vi "CPU_SP_push.vi"(10 "value":u8 format="%02x", 11 "registers":T1 {"P" format="%08b"; "PC" format="%04x"; "SP" format="%02x"; "Y" format="%02x"; "X" format="%02x"; "A" format="%02x"}) -> (3 "registers":T1 {"P" format="%08b"; "PC" format="%04x"; "SP" format="%02x"; "Y" format="%02x"; "X" format="%02x"; "A" format="%02x"})   [LabVIEW 2018]
uses:
  CPU_registers.ctl
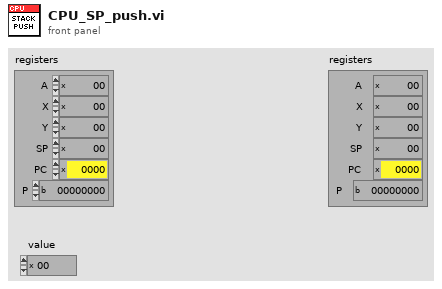
[diagram p1: front panel]
types:
  T1 = typedef "CPU_registers.ctl" = cluster{"A":u8, "X":u8, "Y":u8, "SP":u8, "PC":u16, "P":u8}
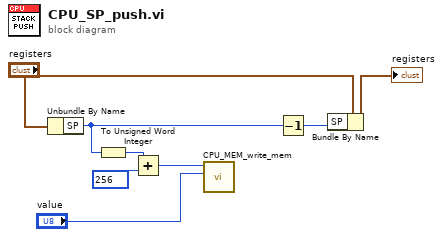
[diagram p0: block diagram]
diagram:
  n1 = Unbundle By Name("registers") -> ("SP"=w4:u8)
  n2 = To Unsigned Word Integer(number=w4) -> (unsigned 16bit integer=w7:u16)
  n3 = Add(x=w7, y=u16 256) -> (x+y=w6:u16)
  n4 = call "CPU_MEM_write_mem.vi"("value"="value", "address"=w6) -> ()  [unwired: 10 in]
  n5 = Decrement(x=w4) -> (x-1=w2:u8)
  n6 = Bundle By Name(cluster="registers", "SP"=w2) -> (→"registers":T1)
